vi "sweep_stimulus.vi"(9 "High corner (Hz)":sgl=150.0 format="%#_3p", 10 "Low corner (Hz)":sgl=5.0 format="%#_3p", 11 "Length (sec)":sgl=5.0 format="%#_3p") -> (3 "Result":sgl[][](array[numeric]))   [LabVIEW 2011]
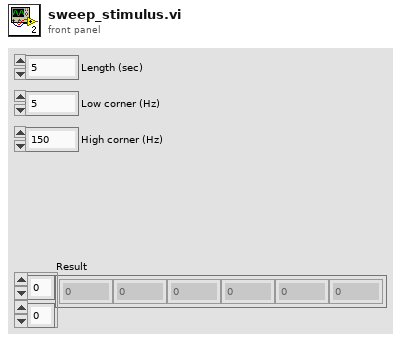
[diagram p1: front panel]
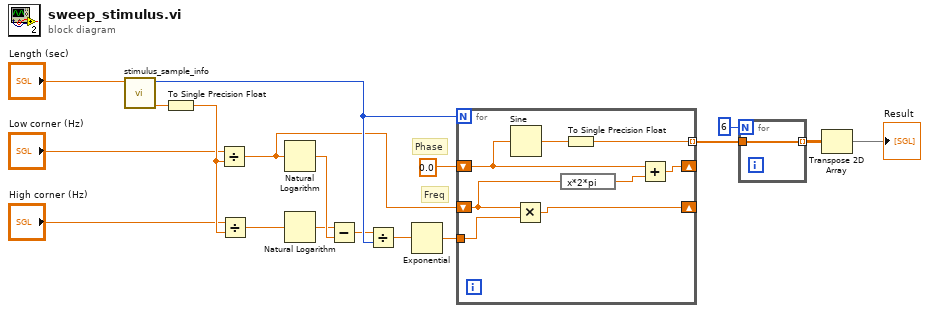
[diagram p0: block diagram]
diagram:
  # "Freq"
  # "Phase"
  n1 = call "stimulus_sample_info.vi"("Length"="Length (sec)") -> ("Sample frequency"=w17:dbl, "Num samples"=w16:i32)  [unwired: 7 in, 2 out]
  n2 = To Single Precision Float(number=w17) -> (single precision float=w18:sgl)
  n3 = Divide(x="Low corner (Hz)", y=w18) -> (x/y=w13:sgl)
  n4 = Divide(x="High corner (Hz)", y=w18) -> (x/y=w14:sgl)
  n5 = Natural Logarithm(1:w13) -> (0:w2:sgl)
  n6 = Natural Logarithm(1:w14) -> (0:w1:sgl)
  n7 = Subtract(x=w1, y=w2) -> (x-y=w3:sgl)
  n8 = Divide(x=w3, y=w16) -> (x/y=w5:sgl)
  n9 = Exponential(1:w5) -> (0:w6:sgl)
  n10 = for {
    N: w16 -> [_]
    shift-right: [w26] -> _
    shift-left: 0.0 ("ln(x)") -> [w25]
    shift-right: [w22] -> _
    shift-left: w13 -> [w23]
    tunnel: w6 -> [w21]
    tunnel: [w19] -> w8 mode=indexing
    n11 = Sine(x=w25) -> (sin(x)=w20:dbl)
    n12 = Multiply(x=w23, y=w21) -> (x*y=w22:sgl)
    n13 = expression code="x*2*pi"(w23) -> (w24:sgl)
    n14 = To Single Precision Float(number=w20) -> (single precision float=w19:sgl)
    n15 = Add(x=w25, y=w24) -> (x+y=w26:dbl)
  }
  n16 = for {
    N: 6 -> [_]
    tunnel: w8 -> [w27]
    tunnel: [w27] -> w9 mode=indexing
  }
  n17 = Transpose 2D Array(2D array=w9) -> (transposed array=→"Result":sgl[][])
